vi "Encoder.vi"() -> ()   [LabVIEW 2019]
uses:
  <vilib>/myRIO/Common/Instrument Driver Framework/myRIO v1.0/Encoder/typedefs/Encoder Signal Mode.ctl
  <vilib>/myRIO/Common/Instrument Driver Framework/myRIO v1.0/UART/vis/myRIO v1.0 Close UART.vi
  <vilib>/myRIO/Common/Instrument Driver Framework/ELVIS III v1.0/Resource Manager/vis/ELVIS III v1.0 Create Configuration List.vi
  <vilib>/Utility/error.llb/Error Cluster From Error Code.vi
  <vilib>/myRIO/Common/Instrument Driver Framework/ELVIS III v1.0/Resource Manager/vis/ELVIS III v1.0 Configure IO.vi
  <vilib>/myRIO/Common/Instrument Driver Framework/ELVIS III v1.0/Resource Manager/vis/ELVIS III v1.0 Unreserve Channel List.vi
  <vilib>/myRIO/Common/Instrument Driver Framework/myRIO v1.0/myRIO v1.0 Close.vi
  <vilib>/myRIO/Common/Instrument Driver Framework/Utilities/vis/FPGA Ref Manager.vi
  <vilib>/myRIO/Common/Instrument Driver Framework/ELVIS III v1.0/ELVIS III v1.0 Reset FPGA.vi
  <vilib>/myRIO/Common/Instrument Driver Framework/myRIO v1.0/IRQ/vis/myRIO v1.0 IRQ Info FGV.vi
  <vilib>/myRIO/Common/Instrument Driver Framework/myRIO v1.0/IRQ/vis/myRIO v1.0 Timer IRQ Info FGV.vi
  <vilib>/myRIO/Common/Instrument Driver Framework/myRIO v1.0/IRQ/vis/myRIO v1.0 ISR Agent.vi
  <vilib>/myRIO/Instrument Drivers/Utilities/vis/Reset Index.vi
  <vilib>/myRIO/Common/Instrument Driver Framework/myRIO v1.0/Resource Manager/vis/myRIO v1.0 Block Write Resource Manager.vi
  <vilib>/myRIO/Instrument Drivers/Utilities/Utilities.lvlib
  <vilib>/myRIO/Instrument Drivers/Onboard IO/Encoder/Encoder.lvlib
panel:
  out "Counter Overflow?":bool
  in  "Reset Counter":bool
  out "Counter Direction":enum16{"Counting Up", "Counting Down"}(ring)
  out "Counter Value":i32
  in  "Stop":bool
  # "ELVIS III Control IO"
  # "긍쯤포"
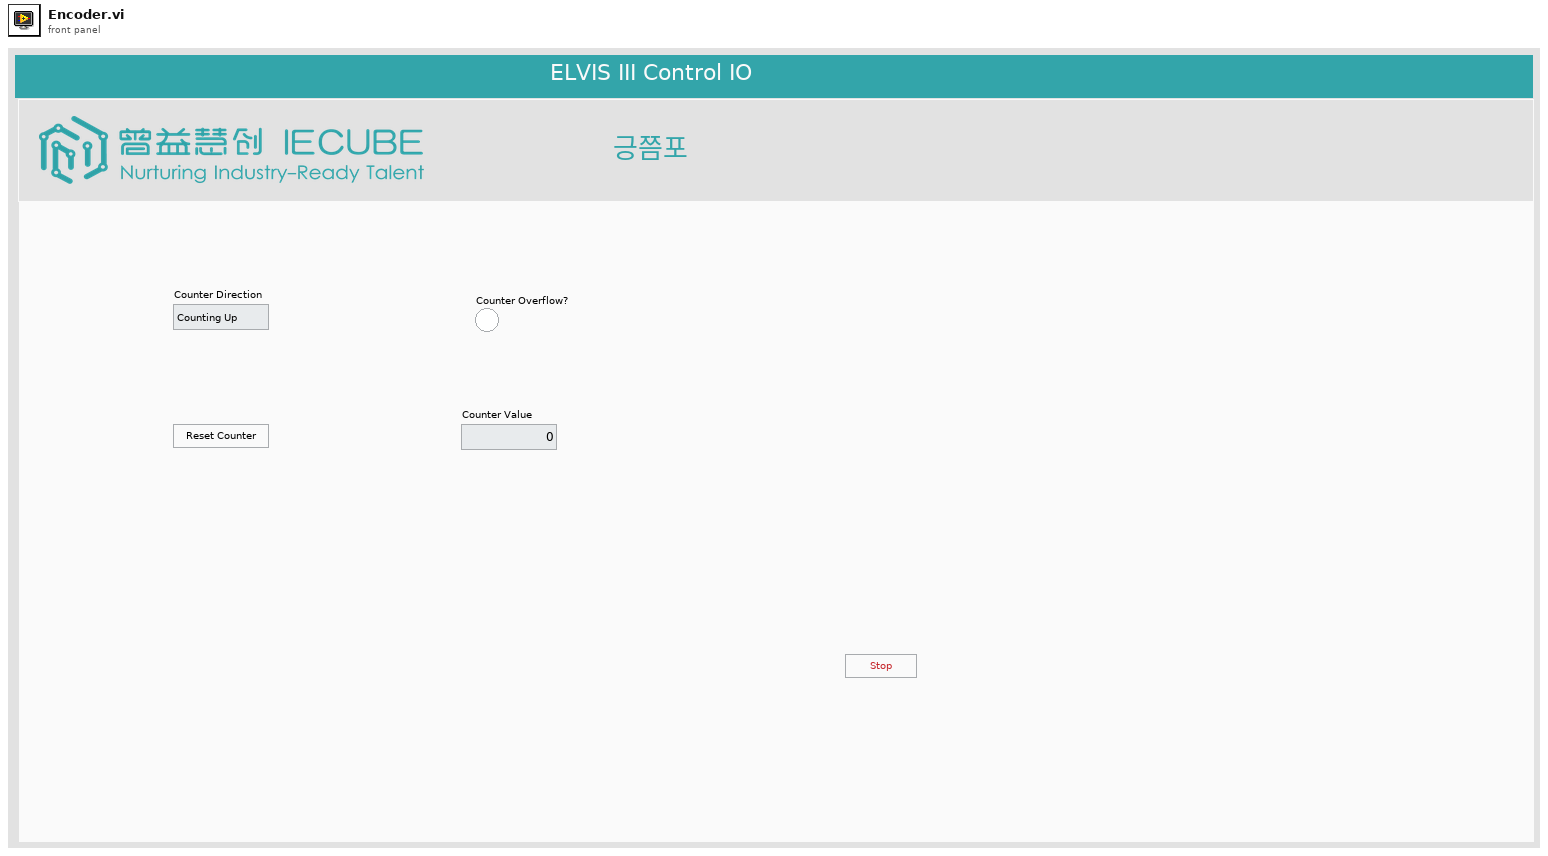
[diagram p1: front panel]
types:
  T1 = typedef "Encoder Signal Mode.ctl" = enum16{"Quadrature phase signal", "Step and direction signal"}
  T2 = typedef "Encoder.lvlib/Encoder Reference.ctl" = cluster{"myRIO Reference":T3, "Encoder Channels Enum":T7}
  T3 = typedef "myRIO Generic Hardware Reference.ctl" = cluster{"myRIO Model":T4, "myRIO Hardware Reference":T5}
  T4 = typedef "Hardware Version Enum.ctl" = enum16{"Unknown", "myRIO-1900", "myRIO-1950", "roboRIO", "NI ELVIS RIO CM", "ELVIS III"}
  T5 = typedef "myRIO v1.0 Reference.ctl" = cluster{"Generic FPGA Reference":T6, "Allow multiple opens":bool}
  T6 = typedef "Generic FPGA Reference.ctl" = refnum<k20>
  T7 = typedef "Encoder Channels Enum.ctl" = enum16{"Not Connected", "C/ENC0", "C/ENC1", "A/ENC", "A/ENC0", "A/ENC1", "A/ENC2", "A/ENC3", "A/ENC4", "A/ENC5", "A/ENC6", "A/ENC7", "A/ENC8", "A/ENC9", "B/ENC", "B/ENC0", "B/ENC1", "B/ENC2", "B/ENC3", "B/ENC4", "B/ENC5", "B/ENC6", "B/ENC7", "B/ENC8", "B/ENC9", "DIO/ENC0", "DIO/ENC1", "DIO/ENC2", "DIO/ENC3", "DIO/ENC4"}
  T8 = typedef "Encoder Count Direction Enum.ctl" = enum16{"Counting Up", "Counting Down"}
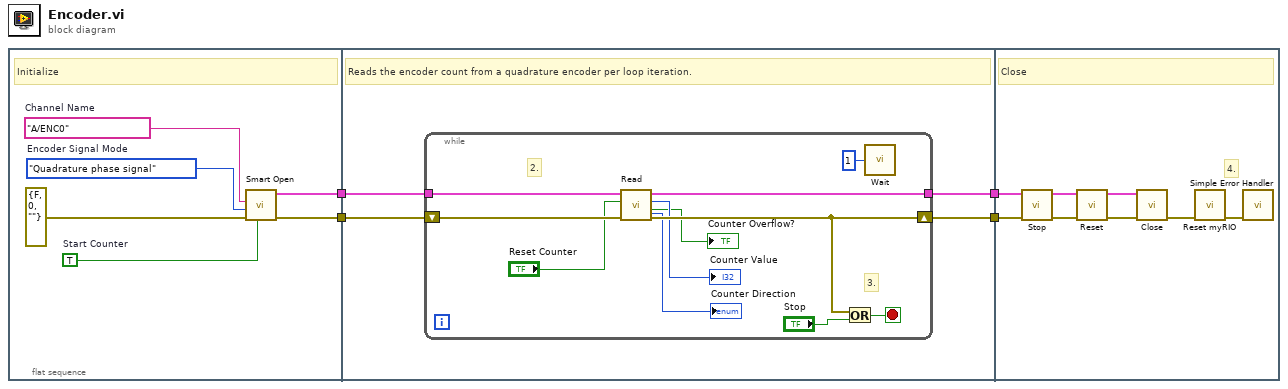
[diagram p0: block diagram]
diagram:
  n1 = flat-sequence {
    tunnel: [w7] -> w3
    tunnel: [w5] -> w2
    tunnel: [w14] -> w4
    tunnel: w3 -> [w13]
    tunnel: w2 -> [w12]
    tunnel: [w11] -> w1
    tunnel: w4 -> [w30]
    tunnel: w1 -> [w32]
    frame #0 {
      w10 = TRUE  # Start Counter
      w9 = Encoder_Signal_Mode."Quadrature phase signal"  # Encoder Signal Mode
      w8 = tag "A/ENC0"  # Channel Name
      # "Initialize"
      n2 = call <vilib>:"Smart Open.vi"("Start Counter"=w10, "error in (no error)"=errorcluster {"status"=FALSE, "code"=0, "source"=""} ("Error In"), "Encoder Signal Mode"=w9, "Channel Name"=w8) -> ("error out"=w7:errorcluster, "Encoder Ref Out"=w5:T2)  [unwired: 6 in]
    }
    frame #1 {
      # "Reads the encoder count from a quadrature encoder per loop iteration."
      n3 = while {
        shift-right: [w21] -> w14
        shift-left: w13 -> [w22]
        tunnel: w12 -> [w20]
        tunnel: [w15] -> w11
        stop <- w25 stop-if-true
        # "3."
        # "2."
        n4 = call <vilib>:"Read.vi"("error in (no error)"=w22, "Reset Counter"="Reset Counter", "Encoder Ref In"=w20) -> ("error out"=w21:errorcluster, "Overflow?"=→"Counter Overflow?":bool, "Counter Value"=→"Counter Value":i32, "Encoder Ref Out"=w15:T2, "Counter Direction"=→"Counter Direction":T8)  [unwired: 4 in]
        n5 = Or(x=w21, y="Stop") -> (x .or. y?=w25:bool)
        n6 = call "Wait"("Count(mSec)"=u32 1) -> ()  [unwired: 1 out]
      }
    }
    frame #2 {
      # "4."
      # "Close"
      n7 = call <vilib>:"Stop.vi"("error in (no error)"=w30, "Encoder Ref In"=w32) -> ("error out"=w29:errorcluster, "Encoder Ref Out"=w31:T2)  [unwired: 8 in]
      n8 = call <vilib>:"Reset.vi"("error in (no error)"=w29, "Encoder Ref In"=w31) -> ("error out"=w28:errorcluster, "Encoder Ref Out"=w26:T2)  [unwired: 8 in]
      n9 = call <vilib>:"Close.vi"("error in (no error)"=w28, "Encoder Ref In"=w26) -> ("error out"=w27:errorcluster)  [unwired: 9 in]
      n10 = call <vilib>:"Reset myRIO.vi"("error in (no error)"=w27) -> ("error out"=w33:errorcluster)  [unwired: 10 in]
      n11 = call <vilib>:"Simple Error Handler.vi"("error in (no error)"=w33) -> ()  [unwired: 4 in, 5 out]
    }
  }
